vi "_06_Sample_qsns_02[17].vi"() -> ()   [LabVIEW 2020]
panel:
  out "Numeric 4":i32
  out "Array":dbl[](array[numeric])
  out "Numeric 3":i32
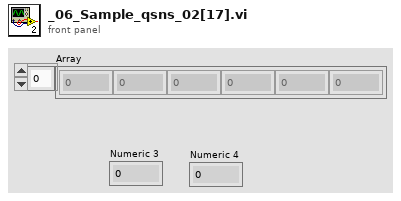
[diagram p1: front panel]
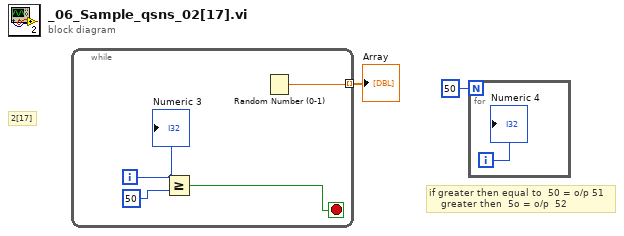
[diagram p0: block diagram]
diagram:
  # "if greater then equal to  50 = o/p 51\n    greater then  5o = o/p  52"
  # "2[17]"
  n1 = while {
    tunnel: [w6] -> w2 mode=indexing
    i -> [w5]
    stop <- w3 stop-if-true
    n2 = Greater Or Equal?(x=w5, y=50) -> (x >= y?=w3:bool)
    n3 = Random Number (0-1)() -> (number: 0 to 1=w6:dbl)
    "Numeric 3" <- w5
  }
  "Array" <- w2
  n4 = for {
    N: 50 -> [_]
    i -> [w7]
    "Numeric 4" <- w7
  }
